vi "HW_Init_2.vi"(8 "error in":errorcluster, 9 "Target FPS":T1, 10 "Close port? (F)":bool, 11 "VISA resource name":refnum<visa-resource-name>="Tracker") -> (0 "error out":errorcluster, 1 "FPS status":i32=80, 2 "Instrument OK?":bool, 3 "VISA resource name out":refnum<visa-resource-name>, 4 "Sync mode status":string, 5 "Sensor board size":string, 7 "FW version information":string)   [LabVIEW 2018]
uses:
  Controls/CTL_Acquisition_speed_selector.ctl
  <vilib>/Utility/error.llb/DialogType.ctl
  <vilib>/Instr/_visa.llb/VISA Set IO Buffer Mask.ctl
  <vilib>/Instr/_visa.llb/VISA Flush IO Buffer Mask.ctl
  <vilib>/Instr/_visa.llb/VISA Configure Serial Port (Instr).vi
panel:
  out "Poll Sync mode status":u32
  in  "FPS setup request":i32=80
  out "Sensors response":string
  out "Poll Port data status":u32
  out "Port data status":i32=1
  out "Latest Poll results (before implemented adjustments)":string="P\r\nI am alive!\r\nA1454 OK!\r\nBinary mode ON\r\nCoordinate mode ON\r\nMatrix mode OFF\r\nFPS target=80\r\nExternal USART status: 0\r\nLed status: 1\r\nPort data status: 1\r\nIOS: 1 = 0, 2 = 0 3 = 0, 4 = 0\r\nOK\r\n"
  out "Poll Binary":u32
  out "Poll Matrix":u32
  out "Poll Coord":u32
  out "Poll FPS":u32
  out "Matrix mode status":string="OFF"
  out "Coordinate mode status":string="ON"
  out "Binary mode status":string="ON"
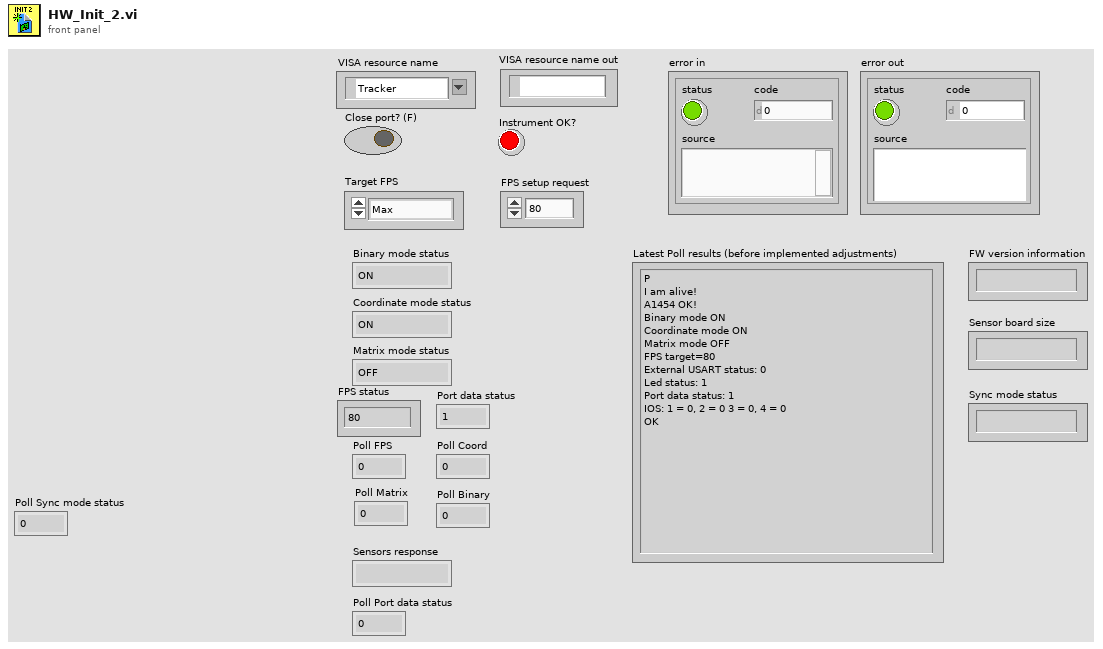
[diagram p1: front panel]
types:
  T1 = typedef "CTL_Acquisition_speed_selector.ctl" = enum16{"Max", "High stability", "Eco"}
  T2 = typedef "DialogType.ctl" = u16
  T3 = typedef "VISA Set IO Buffer Mask.ctl" = u16
  T4 = typedef "VISA Flush IO Buffer Mask.ctl" = u16
  T5 = cluster{"Matrix mode status":string, "Coordinate mode status":string, "Binary mode status":string, "Sensors response":string, "FPS status":i32, "Port data status":i32}
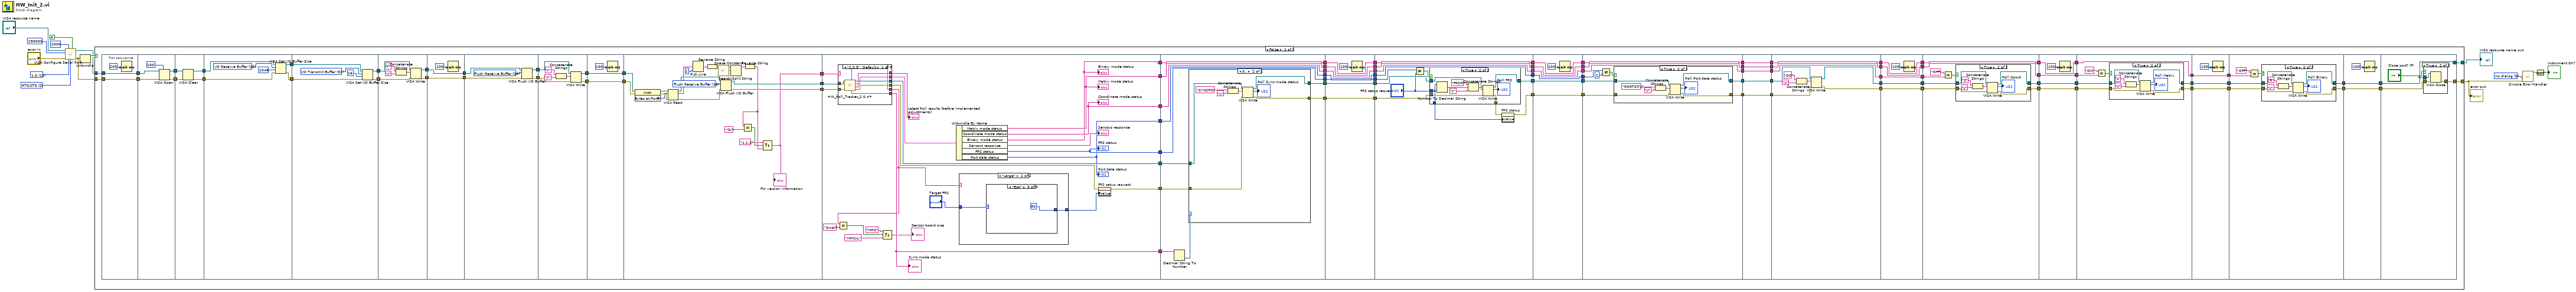
[diagram p0: block diagram]
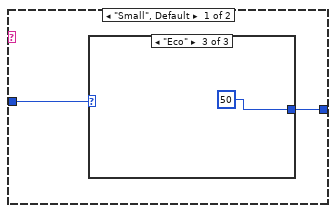
[diagram p2: hidden frame]
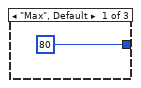
[diagram p3: hidden frame]
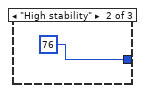
[diagram p4: hidden frame]
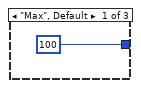
[diagram p5: hidden frame]
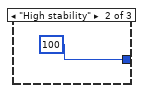
[diagram p6: hidden frame]
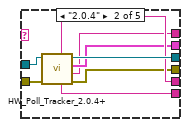
[diagram p7: hidden frame]
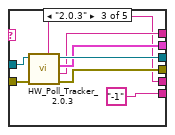
[diagram p8: hidden frame]
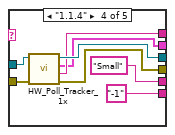
[diagram p9: hidden frame]
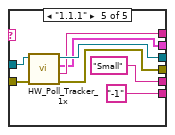
[diagram p10: hidden frame]
diagram:
  w2 = u16 10 items=["1.0"=10, "1.5"=15, "2.0"=20] ("stop bits (10: 1 bit)")
  w4 = T2 0 items=["no dialog", "OK message", "continue or stop message", "OK message + warnings", "continue/stop + warnings"] ("type of dialog (OK msg:1)")
  w9 = u16 2 items=["None", "XON/XOFF", "RTS/CTS", "XON/XOFF & RTS/CTS", "DTR/DSR", "XON/XOFF & DTR/DSR"] ("flow control (0:none)")
  n1 = call-poly "VISA Configure Serial Port"("VISA resource name"="VISA resource name", "timeout (10sec)"=u32 2000, "Enable Termination\nChar (T)"=FALSE ("Enable Termination\nChar (T)"), "baud rate (9600)"=u32 256000, "error in (no error)"="error in", "stop bits (10: 1 bit)"=w2, "flow control (0:none)"=w9) -> ("VISA resource name out"=w8:refnum<visa-resource-name>, "error out"=w11:errorcluster)  [unwired: 7 in]
  n2 = Unbundle(w11) -> ("status"=w10:bool)  [unwired: 2 out]
  n3 = case shown="False" w10 {
    tunnel: w8 -> [w83 w435]
    tunnel: w11 -> [w82 w436]
    tunnel: [w69 w436] -> w7
    tunnel: [w68 w435] -> w1
    frame False {
      n4 = flat-sequence {
        tunnel: [w116] -> w114
        tunnel: [w115] -> w113
        tunnel: w83 -> [w116]
        tunnel: w82 -> [w115]
        tunnel: w114 -> [w120]
        tunnel: [w119] -> w111
        tunnel: w113 -> [w122]
        tunnel: [w121] -> w112
        tunnel: w112 -> [w125]
        tunnel: w111 -> [w126]
        tunnel: [w124] -> w110
        tunnel: [w123] -> w109
        tunnel: [w127] -> w107
        tunnel: [w132] -> w108
        tunnel: w110 -> [w128]
        tunnel: w109 -> [w130]
        tunnel: w108 -> [w136]
        tunnel: [w135] -> w61
        tunnel: w107 -> [w134]
        tunnel: [w133] -> w60
        tunnel: w61 -> [w142]
        tunnel: [w140] -> w57
        tunnel: w60 -> [w141]
        tunnel: [w139] -> w55
        tunnel: w57 -> [w148]
        tunnel: [w148] -> w56
        tunnel: w55 -> [w147]
        tunnel: [w147] -> w54
        tunnel: w56 -> [w151]
        tunnel: [w150] -> w59
        tunnel: w54 -> [w153]
        tunnel: [w152] -> w58
        tunnel: w59 -> [w156]
        tunnel: w58 -> [w157]
        tunnel: [w155] -> w67
        tunnel: [w154] -> w66
        tunnel: w67 -> [w163]
        tunnel: [w163] -> w65
        tunnel: w66 -> [w162]
        tunnel: [w162] -> w63
        tunnel: w65 -> [w180]
        tunnel: [w178] -> w64
        tunnel: w63 -> [w181]
        tunnel: [w176] -> w62
        tunnel: [w165] -> w53
        tunnel: [w194] -> w44
        tunnel: [w207] -> w45
        tunnel: w64 -> [w205]
        tunnel: [w198] -> w42
        tunnel: [w201] -> w40
        tunnel: [w202] -> w38
        tunnel: [w200] -> w36
        tunnel: [w197] -> w34
        tunnel: w62 -> [w204]
        tunnel: w53 -> [w196]
        tunnel: [w193] -> w31
        tunnel: w45 -> [w263]
        tunnel: w44 -> [w261]
        tunnel: [w260] -> w43
        tunnel: w42 -> [w268]
        tunnel: [w268] -> w41
        tunnel: w40 -> [w267]
        tunnel: [w267] -> w39
        tunnel: w38 -> [w266]
        tunnel: [w266] -> w37
        tunnel: w36 -> [w265]
        tunnel: [w265] -> w35
        tunnel: w34 -> [w264]
        tunnel: [w264] -> w33
        tunnel: [w262] -> w32
        tunnel: w31 -> [w259]
        tunnel: [w286] -> w52
        tunnel: w43 -> [w285]
        tunnel: [w285] -> w51
        tunnel: w41 -> [w284]
        tunnel: [w284] -> w50
        tunnel: w39 -> [w283]
        tunnel: [w283] -> w49
        tunnel: w37 -> [w282]
        tunnel: [w282] -> w48
        tunnel: w35 -> [w281]
        tunnel: [w281] -> w47
        tunnel: w33 -> [w280]
        tunnel: [w280] -> w46
        tunnel: w32 -> [w286]
        tunnel: w52 -> [w297]
        tunnel: [w295] -> w106
        tunnel: w51 -> [w296]
        tunnel: [w287] -> w105
        tunnel: w50 -> [w298]
        tunnel: [w294] -> w104
        tunnel: w49 -> [w294]
        tunnel: [w293] -> w103
        tunnel: w48 -> [w293]
        tunnel: [w292] -> w102
        tunnel: w47 -> [w292]
        tunnel: w46 -> [w291]
        tunnel: [w291] -> w70
        tunnel: w106 -> [w319]
        tunnel: [w319] -> w81
        tunnel: w105 -> [w318]
        tunnel: [w318] -> w80
        tunnel: [w316] -> w79
        tunnel: w104 -> [w316]
        tunnel: [w315] -> w78
        tunnel: w103 -> [w315]
        tunnel: [w314] -> w77
        tunnel: w102 -> [w314]
        tunnel: [w313] -> w71
        tunnel: w70 -> [w313]
        tunnel: w81 -> [w324]
        tunnel: [w323] -> w76
        tunnel: w80 -> [w326]
        tunnel: [w325] -> w75
        tunnel: w79 -> [w329]
        tunnel: [w329] -> w74
        tunnel: w78 -> [w328]
        tunnel: [w328] -> w73
        tunnel: w77 -> [w327]
        tunnel: [w327] -> w72
        tunnel: w71 -> [w321]
        tunnel: w76 -> [w344]
        tunnel: [w344] -> w30
        tunnel: w75 -> [w343]
        tunnel: [w343] -> w29
        tunnel: w74 -> [w342]
        tunnel: [w342] -> w28
        tunnel: w73 -> [w341]
        tunnel: [w341] -> w27
        tunnel: w72 -> [w340]
        tunnel: [w340] -> w26
        tunnel: w30 -> [w348]
        tunnel: [w347] -> w25
        tunnel: w29 -> [w346]
        tunnel: [w345] -> w23
        tunnel: w28 -> [w354]
        tunnel: [w354] -> w21
        tunnel: w27 -> [w353]
        tunnel: [w353] -> w19
        tunnel: w26 -> [w352]
        tunnel: [w352] -> w17
        tunnel: w25 -> [w360]
        tunnel: [w360] -> w24
        tunnel: w23 -> [w359]
        tunnel: [w359] -> w22
        tunnel: w21 -> [w358]
        tunnel: [w358] -> w20
        tunnel: w19 -> [w357]
        tunnel: [w357] -> w18
        tunnel: w17 -> [w356]
        tunnel: [w356] -> w16
        tunnel: w24 -> [w368]
        tunnel: [w366] -> w101
        tunnel: w22 -> [w367]
        tunnel: [w363] -> w100
        tunnel: w20 -> [w365]
        tunnel: w18 -> [w362]
        tunnel: [w362] -> w99
        tunnel: w16 -> [w361]
        tunnel: [w361] -> w98
        tunnel: w101 -> [w384]
        tunnel: [w384] -> w97
        tunnel: w100 -> [w383]
        tunnel: [w383] -> w96
        tunnel: [w381] -> w95
        tunnel: w99 -> [w381]
        tunnel: [w380] -> w94
        tunnel: w98 -> [w380]
        tunnel: w97 -> [w390]
        tunnel: [w388] -> w93
        tunnel: w96 -> [w389]
        tunnel: [w387] -> w92
        tunnel: w95 -> [w386]
        tunnel: w94 -> [w385]
        tunnel: [w385] -> w91
        tunnel: w93 -> [w406]
        tunnel: [w406] -> w90
        tunnel: w92 -> [w405]
        tunnel: [w405] -> w89
        tunnel: [w403] -> w88
        tunnel: w91 -> [w403]
        tunnel: w90 -> [w411]
        tunnel: [w409] -> w87
        tunnel: w89 -> [w410]
        tunnel: [w408] -> w86
        tunnel: w88 -> [w407]
        tunnel: w87 -> [w426]
        tunnel: [w426] -> w85
        tunnel: [w425] -> w84
        tunnel: w86 -> [w425]
        tunnel: w85 -> [w427]
        tunnel: w84 -> [w430]
        tunnel: [w428] -> w69
        tunnel: [w427] -> w68
        frame #0 {
          n5 = Wait (ms)(milliseconds to wait=u32 200) -> ()  [unwired: 1 out]
        }
        frame #1 {
          n6 = VISA Open(timeout (0)=u32 100 ("VISA Open timeout (0)"), error in (no error)=w122, VISA resource name=w120) -> (VISA resource name=w119:refnum<visa-resource-name>, error out=w121:errorcluster)  [unwired: 2 in]
        }
        frame #2 {
          n7 = VISA Clear(VISA resource name=w126, error in (no error)=w125) -> (VISA resource name out=w123:refnum<visa-resource-name>, error out=w124:errorcluster)
        }
        frame #3 {
          w129 = T3 16 items=["I/O Receive Buffer"=16, "I/O Transmit Buffer"=32, "I/O Receive and Transmit Buffer"=48] ("Mask")
          n8 = VISA Set I/O Buffer Size(VISA resource name=w130, mask (16)=w129, size (4096)=u32 2048, error in (no error)=w128) -> (VISA resource name out=w132:refnum<visa-resource-name>, error out=w127:errorcluster)
        }
        frame #4 {
          w137 = T3 32 items=["I/O Receive Buffer"=16, "I/O Transmit Buffer"=32, "I/O Receive and Transmit Buffer"=48] ("Mask")
          n9 = VISA Set I/O Buffer Size(VISA resource name=w136, mask (16)=w137, size (4096)=u32 16, error in (no error)=w134) -> (VISA resource name out=w135:refnum<visa-resource-name>, error out=w133:errorcluster)
        }
        frame #5 {
          n10 = Concatenate Strings("T" ("write buffer"), "\r") -> (w143:string)
          n11 = VISA Write(VISA resource name=w142, write buffer=w143, error in (no error)=w141) -> (VISA resource name out=w140:refnum<visa-resource-name>, error out=w139:errorcluster)  [unwired: 1 out]
        }
        frame #6 {
          n12 = Wait (ms)(milliseconds to wait=u32 100) -> ()  [unwired: 1 out]
        }
        frame #7 {
          w149 = T4 16 items=["Flush Receive Buffer"=16, "Write Transmit Buffer to Device"=32, "Flush Receive Buffer (No I/O)"=64, "Flush Transmit Buffer"=128] ("Mask")
          n13 = VISA Flush I/O Buffer(VISA resource name=w151, mask (16)=w149, error in (no error)=w153) -> (VISA resource name out=w150:refnum<visa-resource-name>, error out=w152:errorcluster)
        }
        frame #8 {
          n14 = Concatenate Strings("V" ("write buffer"), "\r") -> (w158:string)
          n15 = VISA Write(VISA resource name=w156, write buffer=w158, error in (no error)=w157) -> (VISA resource name out=w154:refnum<visa-resource-name>, error out=w155:errorcluster)  [unwired: 1 out]
        }
        frame #9 {
          n16 = Wait (ms)(milliseconds to wait=u32 100) -> ()  [unwired: 1 out]
        }
        frame #10 {
          w175 = T4 16 items=["Flush Receive Buffer"=16, "Write Transmit Buffer to Device"=32, "Flush Receive Buffer (No I/O)"=64, "Flush Transmit Buffer"=128] ("Mask")
          n17 = property class="Instr"(reference=w181, error in=w180) -> (reference out=w184:refnum<visa-resource-name>, error out=w183:errorcluster, "Bytes at Port"=w182:u32)
          n18 = VISA Read(VISA resource name=w184, byte count=w182, error in (no error)=w183) -> (VISA resource name out=w177:refnum<visa-resource-name>, read buffer=w174:string, error out=w179:errorcluster)  [unwired: 1 out]
          n19 = Pick Line(multi-line string=w174, line index=1) -> (output string=w172:string)  [unwired: 1 in]
          n20 = Reverse String(1:w172) -> (0:w171:string)
          n21 = call <vilib>:"Space Constant.vi"() -> ("String"=w170:string)
          n22 = VISA Flush I/O Buffer(VISA resource name=w177, mask (16)=w175, error in (no error)=w179) -> (VISA resource name out=w176:refnum<visa-resource-name>, error out=w178:errorcluster)
          n23 = Search/Split String(string=w171, search string/char (-)=w170) -> (substring before match=w169:string)  [unwired: 1 in, 2 out]
          n24 = Reverse String(1:w169) -> (0:w166:string)
          n25 = Equal?(x=w166, y="(b)") -> (x = y?=w167:bool)
          n26 = Select(t="1.1.1", s=w167, f=w166) -> (s? t:f=w165:string)
          "FW version information" <- w165
        }
        frame #11 {
          n27 = case shown="\"2.0.5\", Default" w196 {
            tunnel: [w223 w231 w238 w249 w257] -> w207
            tunnel: [w220 w228 w236 w248 w256] -> w206
            tunnel: w205 -> [w224 w232 w241 w247 w255]
            tunnel: w204 -> [w225 w233 w239 w246 w254]
            tunnel: [w219 w227 w240 w245 w253] -> w195
            tunnel: [w221 w229 w237 w244 w252] -> w203
            tunnel: [w222 w230 w235 "Small" "Small"] -> w187
            tunnel: [w218 w226 "-1" ("Sync mode status") "-1" ("Sync mode status") "-1" ("Sync mode status")] -> w193
            frame "2.0.5", Default {
              n28 = call "HW_Poll_Tracker_2.0.4+.vi"("error in"=w224, "VISA resource name in"=w225) -> ("error out"=w219:errorcluster, "Read buffer"=w220:string, "Parameters output"=w221:T5, "VISA resource name out"=w223:refnum<visa-resource-name>, "Sync mode status"=w218:string, "Sensor board size"=w222:string)  [unwired: 4 in]
            }
            frame "2.0.4" {
              n29 = call "HW_Poll_Tracker_2.0.4+.vi"("error in"=w232, "VISA resource name in"=w233) -> ("error out"=w227:errorcluster, "Read buffer"=w228:string, "Parameters output"=w229:T5, "VISA resource name out"=w231:refnum<visa-resource-name>, "Sync mode status"=w226:string, "Sensor board size"=w230:string)  [unwired: 4 in]
            }
            frame "2.0.3" {
              n30 = call "HW_Poll_Tracker_2.0.3.vi"("error in"=w241, "VISA resource name in"=w239) -> ("error out"=w240:errorcluster, "Read buffer"=w236:string, "Parameters output"=w237:T5, "VISA resource name out"=w238:refnum<visa-resource-name>, "Sensor board size"=w235:string)  [unwired: 5 in]
            }
            frame "1.1.4" {
              n31 = call "HW_Poll_Tracker_1x.vi"("error in"=w247, "VISA resource name in"=w246) -> ("error out"=w245:errorcluster, "Read buffer"=w248:string, "Parameters output"=w244:T5, "VISA resource name out"=w249:refnum<visa-resource-name>)  [unwired: 6 in]
            }
            frame "1.1.1" {
              n32 = call "HW_Poll_Tracker_1x.vi"("error in"=w255, "VISA resource name in"=w254) -> ("error out"=w253:errorcluster, "Read buffer"=w256:string, "Parameters output"=w252:T5, "VISA resource name out"=w257:refnum<visa-resource-name>)  [unwired: 6 in]
            }
          }
          "Latest Poll results (before implemented adjustments)" <- w206
          "Sync mode status" <- w193
          n33 = Equal?(x=w187, y="Small") -> (x = y?=w190:bool)
          n34 = Select(t="MHC" ("x"), s=w190, f="MHC-L") -> (s? t:f=→"Sensor board size":string)
          n35 = Unbundle By Name(w203) -> ("Matrix mode status"=w202:string, "Coordinate mode status"=w201:string, "Binary mode status"=w200:string, "Sensors response"=→"Sensors response":string, "FPS status"=w198:i32, "Port data status"=w197:i32)
          "Binary mode status" <- w200
          "Coordinate mode status" <- w201
          "Matrix mode status" <- w202
          "FPS status" <- w198
          "Port data status" <- w197
          n36 = case shown="\"Large\"" w187 {
            tunnel: "Target FPS" -> [w209 w214]
            tunnel: [w208 w213] -> w191
            frame "Small", Default {
              n37 = case shown="\"Eco\"" w209 {
                tunnel: [80 76 50] -> w208
                frame "Max", Default {
                }
                frame "High stability" {
                }
                frame "Eco" {
                }
              }
            }
            frame "Large" {
              n38 = case shown="\"Eco\"" w214 {
                tunnel: [100 100 50] -> w213
                frame "Max", Default {
                }
                frame "High stability" {
                }
                frame "Eco" {
                }
              }
            }
          }
          n39 = property on="FPS setup request" class="DigNum (strict)"(error in=w195, "Value"=w191) -> (error out=w194:errorcluster)  [unwired: 1 in, 1 out]
        }
        frame #12 {
          n40 = Decimal String To Number(string=w259) -> (number=w258:i32)  [unwired: 2 in, 1 out]
          n41 = case shown="0.." w258 {
            tunnel: w263 -> [w270 w276]
            tunnel: w261 -> [w269 w275]
            tunnel: [w269 w274] -> w260
            tunnel: [w270 w273] -> w262
            frame -1, Default {
            }
            frame 0.. {
              n42 = Concatenate Strings("SYNC=0" ("write buffer"), "\r") -> (w278:string)
              n43 = VISA Write(VISA resource name=w276, write buffer=w278, error in (no error)=w275) -> (VISA resource name out=w273:refnum<visa-resource-name>, return count=→"Poll Sync mode status":u32, error out=w274:errorcluster)
            }
          }
        }
        frame #13 {
          n44 = Wait (ms)(milliseconds to wait=u32 100) -> ()  [unwired: 1 out]
        }
        frame #14 {
          n45 = Not Equal?(x=w298, y="FPS setup request") -> (x != y?=w299:bool)
          n46 = case shown="True" w299 {
            tunnel: w297 -> [w302 w309]
            tunnel: w296 -> [w300 w308]
            tunnel: [w302 w307] -> w295
            tunnel: "FPS setup request" -> [w301 w304]
            tunnel: [w301 w304] -> w289
            tunnel: [w300 w303] -> w288
            frame False {
            }
            frame True {
              n47 = Number To Decimal String(number=w304) -> (decimal integer string=w305:string)  [unwired: 1 in]
              n48 = Concatenate Strings("FPS=" ("write buffer"), w305, "\r") -> (w311:string)
              n49 = VISA Write(VISA resource name=w309, write buffer=w311, error in (no error)=w308) -> (VISA resource name out=w307:refnum<visa-resource-name>, return count=→"Poll FPS":u32, error out=w303:errorcluster)
            }
          }
          n50 = property on="FPS status" class="DigNum (strict)"(error in=w288, "Value"=w289) -> (error out=w287:errorcluster)  [unwired: 1 in, 1 out]
        }
        frame #15 {
          n51 = Wait (ms)(milliseconds to wait=u32 100) -> ()  [unwired: 1 out]
        }
        frame #16 {
          n52 = Not Equal?(x=w321, y=1) -> (x != y?=w320:bool)
          n53 = case shown="True" w320 {
            tunnel: w326 -> [w330 w335]
            tunnel: [w330 w334] -> w325
            tunnel: w324 -> [w331 w333]
            tunnel: [w331 w332] -> w323
            frame False {
            }
            frame True {
              n54 = Concatenate Strings("PORTS=1" ("write buffer"), "\r") -> (w337:string)
              n55 = VISA Write(VISA resource name=w333, write buffer=w337, error in (no error)=w335) -> (VISA resource name out=w332:refnum<visa-resource-name>, return count=→"Poll Port data status":u32, error out=w334:errorcluster)
            }
          }
        }
        frame #17 {
        }
        frame #18 {
          n56 = Concatenate Strings("O0" ("write buffer"), "\r") -> (w349:string)
          n57 = VISA Write(VISA resource name=w348, write buffer=w349, error in (no error)=w346) -> (VISA resource name out=w347:refnum<visa-resource-name>, error out=w345:errorcluster)  [unwired: 1 out]
        }
        frame #19 {
          n58 = Wait (ms)(milliseconds to wait=u32 100) -> ()  [unwired: 1 out]
        }
        frame #20 {
          n59 = Equal?(x="OFF", y=w365) -> (x = y?=w369:bool)
          n60 = case shown="True" w369 {
            tunnel: w368 -> [w371 w375]
            tunnel: w367 -> [w370 w374]
            tunnel: [w371 w373] -> w366
            tunnel: [w370 w372] -> w363
            frame False {
            }
            frame True {
              n61 = Concatenate Strings("C" ("write buffer"), "\r") -> (w377:string)
              n62 = VISA Write(VISA resource name=w375, write buffer=w377, error in (no error)=w374) -> (VISA resource name out=w373:refnum<visa-resource-name>, return count=→"Poll Coord":u32, error out=w372:errorcluster)
            }
          }
        }
        frame #21 {
          n63 = Wait (ms)(milliseconds to wait=u32 100) -> ()  [unwired: 1 out]
        }
        frame #22 {
          n64 = Equal?(x="ON", y=w386) -> (x = y?=w392:bool)
          n65 = case shown="True" w392 {
            tunnel: w390 -> [w394 w398]
            tunnel: w389 -> [w393 w397]
            tunnel: [w394 w396] -> w388
            tunnel: [w393 w395] -> w387
            frame False {
            }
            frame True {
              n66 = Concatenate Strings("L" ("write buffer"), "\r") -> (w400:string)
              n67 = VISA Write(VISA resource name=w398, write buffer=w400, error in (no error)=w397) -> (VISA resource name out=w396:refnum<visa-resource-name>, return count=→"Poll Matrix":u32, error out=w395:errorcluster)
            }
          }
        }
        frame #23 {
          n68 = Wait (ms)(milliseconds to wait=u32 100) -> ()  [unwired: 1 out]
        }
        frame #24 {
          n69 = Equal?(x="OFF", y=w407) -> (x = y?=w413:bool)
          n70 = case shown="True" w413 {
            tunnel: w411 -> [w415 w419]
            tunnel: w410 -> [w414 w418]
            tunnel: [w415 w417] -> w409
            tunnel: [w414 w416] -> w408
            frame False {
            }
            frame True {
              n71 = Concatenate Strings("B" ("write buffer"), "\r") -> (w421:string)
              n72 = VISA Write(VISA resource name=w419, write buffer=w421, error in (no error)=w418) -> (VISA resource name out=w417:refnum<visa-resource-name>, return count=→"Poll Binary":u32, error out=w416:errorcluster)
            }
          }
        }
        frame #25 {
          n73 = Wait (ms)(milliseconds to wait=u32 100) -> ()  [unwired: 1 out]
        }
        frame #26 {
          n74 = case shown="True" "Close port? (F)" {
            tunnel: w430 -> [w431 w434]
            tunnel: [w431 w433] -> w428
            tunnel: w427 -> [_ w432]
            frame False {
            }
            frame True {
              n75 = VISA Close(VISA resource name=w432, error in (no error)=w434) -> (error out=w433:errorcluster)
            }
          }
        }
      }
    }
    frame True {
    }
  }
  "error out" <- w7
  "VISA resource name out" <- w1
  n76 = call <vilib>:"Simple Error Handler.vi"("type of dialog (OK msg:1)"=w4, "error in (no error)"=w7) -> ("error?"=w6:bool)  [unwired: 3 in, 4 out]
  n77 = Not(x=w6) -> (.not. x?=→"Instrument OK?":bool)
